vi "ConstellationInit.vi"(8 "Error in":errorcluster, 10 "Active Controllers":cluster{"Status":bool, "Number":dbl}[](array[cluster])=[{"Status"=TRUE, "Number"=0.0}, {"Status"=FALSE, "Number"=1.0}], 11 "USB Ports":refnum<visa-resource-name>[](array[refnum])=["COM8"]) -> (0 "Error out":errorcluster={"status"=TRUE, "code"=-1073807343, "source"="Property Node (arg 1) in VISA Configure Serial Port (Instr).vi->ConstellationInit.vi"}, 1 "Active Boards out":cluster{"Status":bool, "Board":string}[][](array[cluster]), 2 "Active Controllers out":cluster{"Status":bool, "Number":dbl}[](array[cluster])=[{"Status"=TRUE, "Number"=0.0}, {"Status"=FALSE, "Number"=1.0}], 3 "Task out":refnum<visa-resource-name>[](array[refnum]))   [LabVIEW 2012]
uses:
  <vilib>/Instr/_visa.llb/VISA Configure Serial Port (Instr).vi
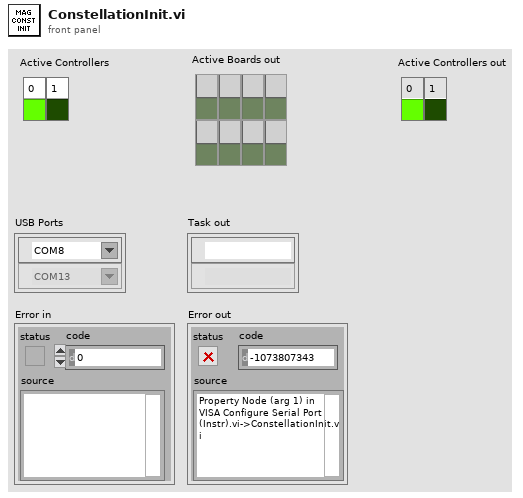
[diagram p1: front panel]
types:
  T1 = enum16{"big-endian, network order", "native, host order", "little-endian"}
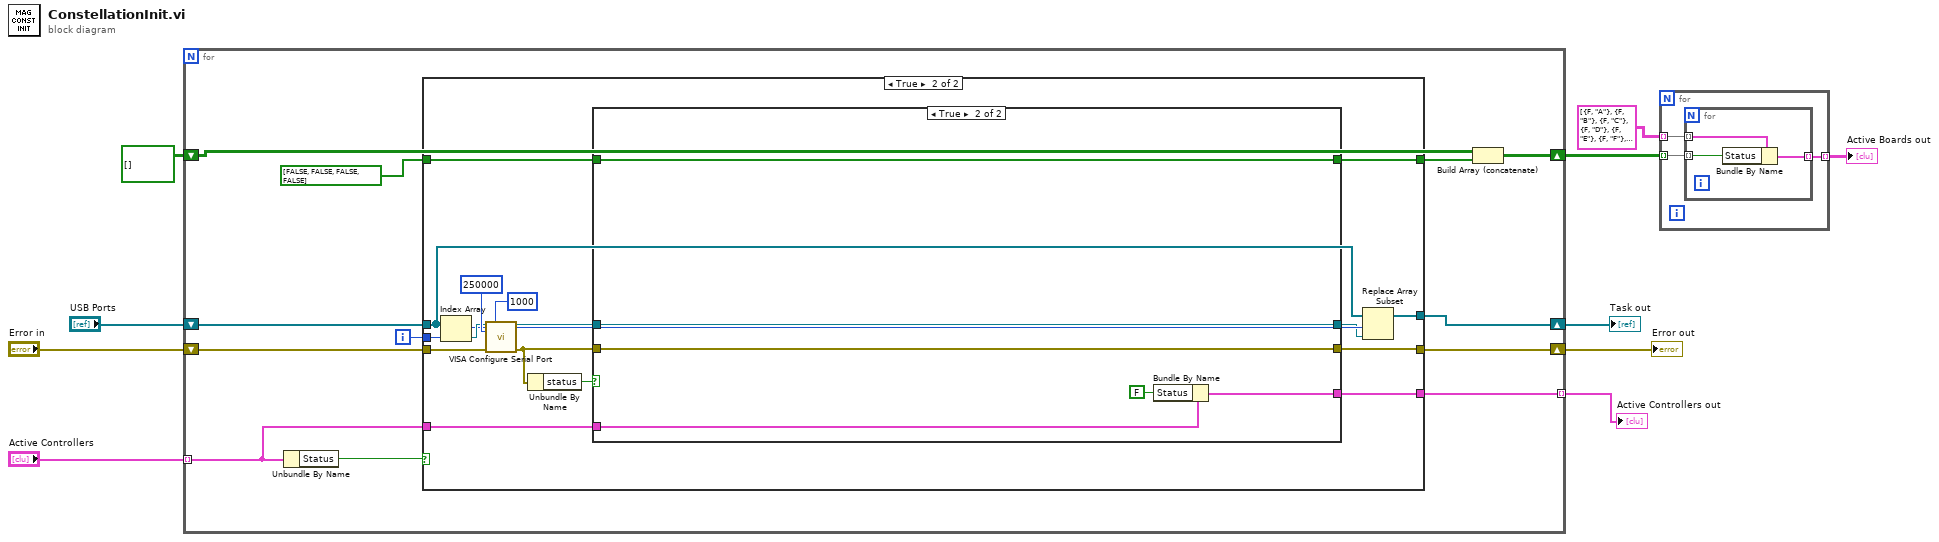
[diagram p0: block diagram]
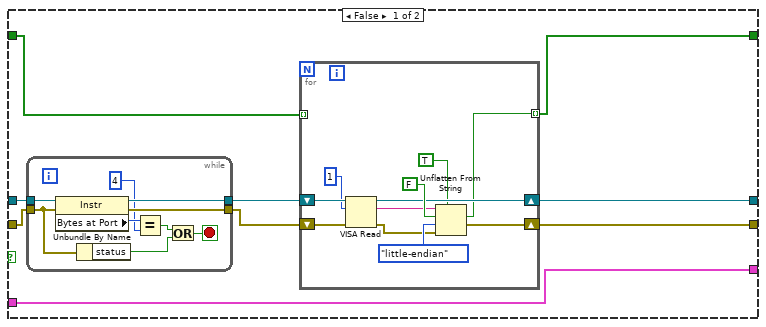
[diagram p3: hidden frame]
diagram:
  n1 = for {
    shift-right: [w21] -> w9
    shift-left: "Error in" -> [w22]
    tunnel: "Active Controllers" -> [w17] mode=indexing
    tunnel: [w16] -> w6 mode=indexing
    shift-right: [w15] -> w5
    shift-left: "USB Ports" -> [w19]
    shift-right: [w12] -> w3
    shift-left: bool[][] [] -> [w11]
    i -> [w18]
    n2 = Unbundle By Name(w17) -> ("Status"=w20:bool)
    n3 = case shown="True" w20 {
      tunnel: w22 -> [w26 w42]
      tunnel: [w26 w38] -> w21
      tunnel: w19 -> [w24 w32]
      tunnel: w18 -> [_ w30]
      tunnel: w17 -> [w25 w34]
      tunnel: [w25 w33] -> w16
      tunnel: [w24 w31] -> w15
      tunnel: [w23 w28] -> w14
      tunnel: bool[] [FALSE, FALSE, FALSE, FALSE] -> [w23 w27]
      frame False {
      }
      frame True {
        n4 = Index Array(array=w32, index=w30) -> (element=w35:refnum<visa-resource-name>)
        n5 = call-poly "VISA Configure Serial Port"("VISA resource name"=w35, "timeout (10sec)"=u32 1000, "baud rate (9600)"=u32 250000, "error in (no error)"=w42) -> ("VISA resource name out"=w41:refnum<visa-resource-name>, "error out"=w37:errorcluster)  [unwired: 10 in]
        n6 = Unbundle By Name(w37) -> ("status"=w36:bool)
        n7 = case shown="True" w36 {
          tunnel: w41 -> [w51 w73]
          tunnel: w37 -> [w50 w77]
          tunnel: [w47 w73] -> w29
          tunnel: [w46 w77] -> w38
          tunnel: w34 -> [w45 w76]
          tunnel: [w45 w74] -> w33
          tunnel: [w44 w72] -> w28
          tunnel: w27 -> [w43 w72]
          frame False {
            n8 = while {
              tunnel: w51 -> [w60]
              tunnel: w50 -> [w57]
              tunnel: [w59] -> w49
              tunnel: [w58] -> w48
              stop <- w55 stop-if-true
              n9 = property class="Instr"(reference=w60, error in=w57) -> (reference out=w59:refnum<visa-resource-name>, error out=w58:errorcluster, "Bytes at Port"=w53:u32)
              n10 = Unbundle By Name(w57) -> ("status"=w56:bool)
              n11 = Equal?(x=w53, y=4) -> (x = y?=w54:bool)
              n12 = Or(x=w54, y=w56) -> (x .or. y?=w55:bool)
            }
            n13 = for {
              shift-right: [w66] -> w47
              shift-left: w49 -> [w71]
              shift-right: [w64] -> w46
              shift-left: w48 -> [w70]
              tunnel: [w61] -> w44 mode=indexing
              tunnel: w43 -> [_] mode=indexing
              n14 = VISA Read(VISA resource name=w71, byte count=u32 1, error in (no error)=w70) -> (VISA resource name out=w66:refnum<visa-resource-name>, read buffer=w67:string, error out=w65:errorcluster)  [unwired: 1 out]
              n15 = Unflatten From String(type=TRUE, binary string=w67, data includes array or string size? (T)=FALSE, byte order (0:big-endian, network order)=T1."little-endian", error in (no error)=w65) -> (value=w61:bool, error out=w64:errorcluster)  [unwired: 1 out]
            }
          }
          frame True {
            n16 = Bundle By Name(cluster=w76, "Status"=FALSE) -> (w74:cluster{"Status":bool, "Number":dbl})
          }
        }
        n17 = Replace Array Subset(array=w32, new element=w29, index=w30) -> (w31:refnum<visa-resource-name>[])
      }
    }
    n18 = Build Array (concatenate)(w11, w14) -> (w12:bool[][])
  }
  "Task out" <- w5
  "Error out" <- w9
  "Active Controllers out" <- w6
  n19 = for {
    tunnel: cluster{"Status":bool, "Board":string}[][] [[{"Status"=FALSE, "Board"="A"}, {"Status"=FALSE, "Board"="B"}, {"Status"=FALSE, "Board"="C"}, {"Status"=FALSE, "Board"="D"}], [{"Status"=FALSE, "Board"="E"}, {"Status"=FALSE, "Board"="F"}, {"Status"=FALSE, "Board"="G"}, {"Status"=FALSE, "Board"="H"}]] ("Active Boards out 2") -> [w80] mode=indexing
    tunnel: w3 -> [w79] mode=indexing
    tunnel: [w78] -> w2 mode=indexing
    n20 = for {
      tunnel: w80 -> [w83] mode=indexing
      tunnel: w79 -> [w82] mode=indexing
      tunnel: [w81] -> w78 mode=indexing
      n21 = Bundle By Name(cluster=w83, "Status"=w82) -> (w81:cluster{"Status":bool, "Board":string})
    }
  }
  "Active Boards out" <- w2
